vi "TimeCalculator.vi"(1 "TimerRegisters":T1={"Tick0"="Tick0", "Tock0"="Tock0", "Tick1"="Tick1", "Tock1"="Tock1", "Tick2"="Tick1", "Tock2"="Tock1", "Tick3"="Tick1", "Tock3"="Tock1", "Tick4"="Tick0", "Tock4"="Tock0", "Tick5"="Tick1", "Tock5"="Tock1", "Tick6"="Tick1", "Tock6"="Tock1", "Tick7"="Tick1", "Tock7"="Tock1"}, 11 "resetMaxTime":bool) -> (4 "Times":u32[](array[numeric]), 6 "MaxTimes":u32[](array[numeric]))   [LabVIEW 2015, in "Timers.lvlib"]
doc: "Calculates the time between the tick and tick VI of a single timer. It also hold the maximum time in a register that can be reset."
uses:
  Timers.lvlib
  TimerRegisters.ctl
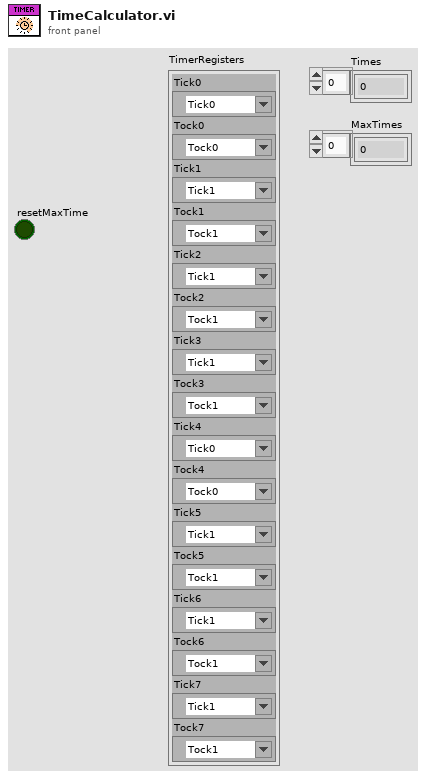
[diagram p1: front panel]
types:
  T1 = typedef "Timers.lvlib/TimerRegisters.ctl" = cluster{"Tick0":refnum<k21>, "Tock0":refnum<k21>, "Tick1":refnum<k21>, "Tock1":refnum<k21>, "Tick2":refnum<k21>, "Tock2":refnum<k21>, "Tick3":refnum<k21>, "Tock3":refnum<k21>, "Tick4":refnum<k21>, "Tock4":refnum<k21>, "Tick5":refnum<k21>, "Tock5":refnum<k21>, "Tick6":refnum<k21>, "Tock6":refnum<k21>, "Tick7":refnum<k21>, "Tock7":refnum<k21>}
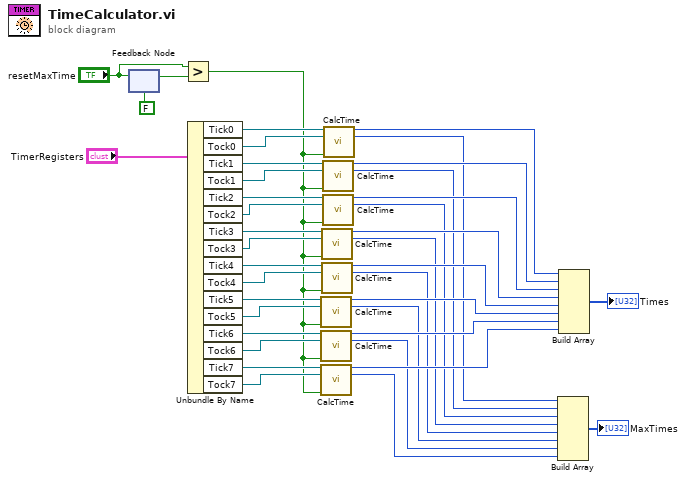
[diagram p0: block diagram]
diagram:
  n1 = feedback-in #1("resetMaxTime") -> ()
  n2 = feedback #1(FALSE ("resetMaxTime")) -> (w3:bool)
  n3 = Greater?(x="resetMaxTime", y=w3) -> (0:w1:bool)
  n4 = Unbundle By Name("TimerRegisters") -> ("Tick0"=w37:refnum<k21>, "Tock0"=w36:refnum<k21>, "Tick1"=w34:refnum<k21>, "Tock1"=w33:refnum<k21>, "Tick2"=w31:refnum<k21>, "Tock2"=w30:refnum<k21>, "Tick3"=w28:refnum<k21>, "Tock3"=w27:refnum<k21>, "Tick4"=w26:refnum<k21>, "Tock4"=w25:refnum<k21>, "Tick5"=w24:refnum<k21>, "Tock5"=w23:refnum<k21>, "Tick6"=w22:refnum<k21>, "Tock6"=w21:refnum<k21>, "Tick7"=w20:refnum<k21>, "Tock7"=w19:refnum<k21>)
  n5 = call "CalcTime.vi"("TickRef"=w24, "TockRef"=w23, "resetMaxTime"=w1) -> ("Time"=w16:u32, "MaxTime"=w8:u32)  [unwired: 11 in]
  n6 = call "CalcTime.vi"("TickRef"=w22, "TockRef"=w21, "resetMaxTime"=w1) -> ("Time"=w15:u32, "MaxTime"=w7:u32)  [unwired: 11 in]
  n7 = call "CalcTime.vi"("TickRef"=w20, "TockRef"=w19, "resetMaxTime"=w1) -> ("Time"=w14:u32, "MaxTime"=w6:u32)  [unwired: 11 in]
  n8 = call "CalcTime.vi"("TickRef"=w28, "TockRef"=w27, "resetMaxTime"=w1) -> ("Time"=w18:u32, "MaxTime"=w10:u32)  [unwired: 11 in]
  n9 = call "CalcTime.vi"("TickRef"=w26, "TockRef"=w25, "resetMaxTime"=w1) -> ("Time"=w17:u32, "MaxTime"=w9:u32)  [unwired: 11 in]
  n10 = call "CalcTime.vi"("TickRef"=w34, "TockRef"=w33, "resetMaxTime"=w1) -> ("Time"=w32:u32, "MaxTime"=w12:u32)  [unwired: 11 in]
  n11 = call "CalcTime.vi"("TickRef"=w31, "TockRef"=w30, "resetMaxTime"=w1) -> ("Time"=w29:u32, "MaxTime"=w11:u32)  [unwired: 11 in]
  n12 = call "CalcTime.vi"("TickRef"=w37, "TockRef"=w36, "resetMaxTime"=w1) -> ("Time"=w35:u32, "MaxTime"=w13:u32)  [unwired: 11 in]
  n13 = Build Array(w13, w12, w11, w10, w9, w8, w7, w6) -> (→"MaxTimes":u32[])
  n14 = Build Array(w35, w32, w29, w18, w17, w16, w15, w14) -> (→"Times":u32[])
